vi "WT1600 Main.vi"() -> ()   [LabVIEW 2013, in "WT1600.lvlib"]
uses:
  WT1600/WT1600.lvlib
  <vilib>/ActorFramework/Message Queue/Message Queue.lvclass
  <vilib>/ActorFramework/Actor/Actor.lvclass
  <vilib>/ActorFramework/Stop Msg/Stop Msg.lvclass
  WT1600/WT1600/WT1600.lvclass
panel:
  out "error out":errorcluster
  in  "WT1600.lvlib:WT1600.lvclass":refnum<class "WT1600.lvclass">
  in  "Stop Button":bool
  in  "WT1600 vISA":refnum<visa-resource-name>="GPIB0::10::INSTR"
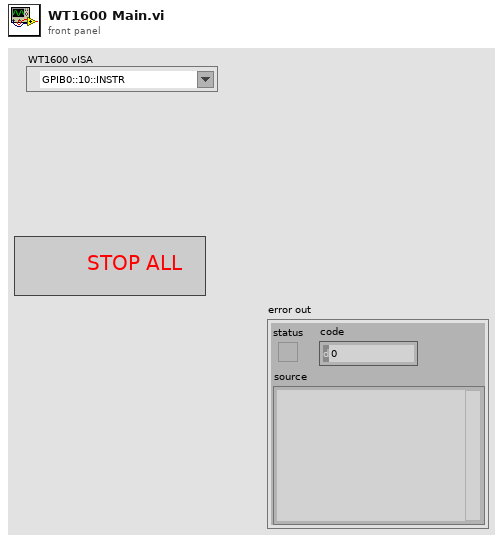
[diagram p1: front panel]
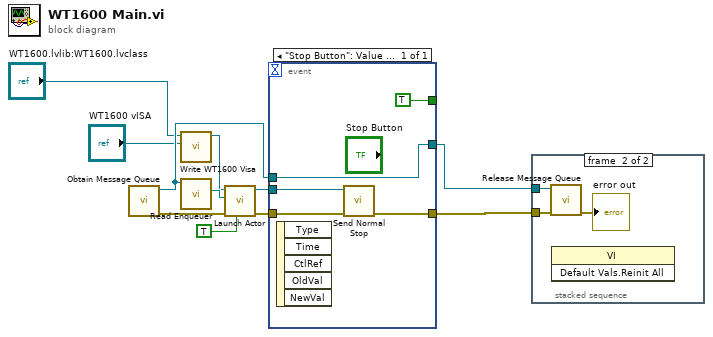
[diagram p0: block diagram]
diagram:
  n1 = call <vilib>:"Obtain Message Queue.vi"() -> ("error out"=w7:errorcluster, "Message Queue"=w9:refnum<class "Message Queue.lvclass">)  [unwired: 10 in]
  n2 = call "Write WT1600 Visa.vi"("WT1600 VISA"="WT1600 vISA", "WT1600 in"="WT1600.lvlib:WT1600.lvclass") -> ("WT1600 out"=w3:refnum<class "WT1600.lvclass">)  [unwired: 8 in, 1 out]
  n3 = call <vilib>:"Read Enqueuer.vi"("Message Queue"=w9) -> ("Message Enqueuer"=w10:refnum<class "Message Enqueuer.lvclass">)  [unwired: 10 in]
  n4 = call <vilib>:"Launch Actor.vi"("Open Actor Core front panel? (F)"=TRUE, "error in (no error)"=w7, "Actor-to-Caller Enqueuer"=w10, "Actor"=w3) -> ("error out"=w8:errorcluster, "Caller-To-Actor Enqueuer"=w1:refnum<class "Message Enqueuer.lvclass">)  [unwired: 6 in]
  n5 = event shown="[0] \"Stop Button\": Value Change" {
    selector: _ -> [_]
    dyn-events: _ -> [_]
    timeout: _ -> [_]
    tunnel: w1 -> [w16]
    tunnel: w9 -> [w13]
    tunnel: w8 -> [w15]
    tunnel: [TRUE] -> _
    tunnel: [w13] -> w6
    tunnel: [w12] -> w5
    event "Stop Button": Value Change {
      n6 = event-data() -> ()  [unwired: 1 in, 5 out]
      n7 = call <vilib>:"Send Normal Stop.vi"("error in (no error)"=w15, "Message Enqueuer"=w16) -> ("error out"=w12:errorcluster)  [unwired: 9 in]
    }
  }
  n8 = stacked-sequence {
    tunnel: w6 -> [_ w18]
    tunnel: w5 -> [_ w17]
    frame #0 {
    }
    frame #1 {
      n9 = call <vilib>:"Release Message Queue.vi"("error in (no error)"=w17, "Message Queue"=w18) -> ("error out"=→"error out":errorcluster)  [unwired: 8 in, 1 out]
      n10 = invoke class="VI" method="Default Vals.Reinit All"() -> ()  [unwired: 3 in, 3 out]
    }
  }
